vi "check_data (SubVI).vi"(1 "read buffer":string) -> (8 "buffer out":string, 9 "bool out":bool)   [LabVIEW 2015]
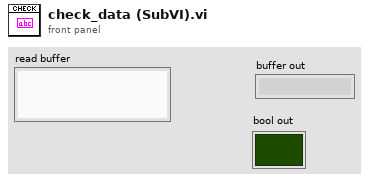
[diagram p1: front panel]
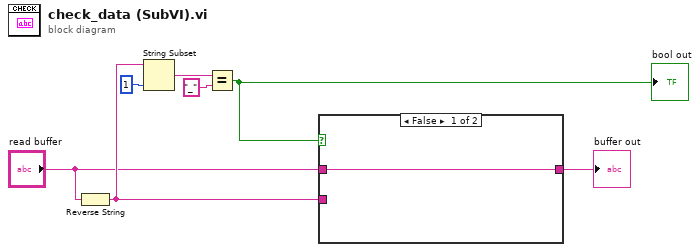
[diagram p0: block diagram]
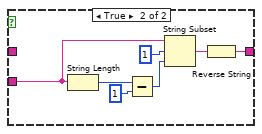
[diagram p2: hidden frame]
diagram:
  n1 = Reverse String(1:"read buffer") -> (0:w3:string)
  n2 = String Subset(string=w3, length (rest)=1 ("length (rest)")) -> (substring=w7:string)  [unwired: 1 in]
  n3 = Equal?(x=w7, y="_") -> (x = y?=w1:bool)
  "bool out" <- w1
  n4 = case shown="False" w1 {
    tunnel: w3 -> [_ w13]
    tunnel: [w8 w9] -> w4
    tunnel: "read buffer" -> [w8 _]
    frame False {
    }
    frame True {
      n5 = String Length(string=w13) -> (length=w15:i32)
      n6 = Subtract(x=w15, y=1) -> (x-y=w11:i32)
      n7 = String Subset(string=w13, offset (0)=1, length (rest)=w11) -> (substring=w10:string)
      n8 = Reverse String(1:w10) -> (0:w9:string)
    }
  }
  "buffer out" <- w4
